vi "Configure.vi"(8 "error in (no error)":errorcluster, 11 "DAQ_QPT_Throlab in":refnum<class "DAQ_QPT_Throlab.lvclass">) -> (0 "error out":errorcluster, 3 "DAQ_QPT_Throlab out":refnum<class "DAQ_QPT_Throlab.lvclass">)   [LabVIEW 2020, in "DAQ_QPT_Throlab.lvlib" / "DAQ_QPT_Throlab.lvclass"]
uses:
  DAQ_QPT_Throlab.lvclass
  E:/Development/DevHardSoftware/MMicroscopyAF/Model/HAL Layer/Component/Device/Device/Device.lvclass
  DAQ_QPT_Throlab.lvclass/DAQ_QPT_Throlab.ctl
  HAL Layer/Component/DAQ/DAQ/DAQ.lvclass
  HAL Layer/Component/Device/Device/Device.lvclass
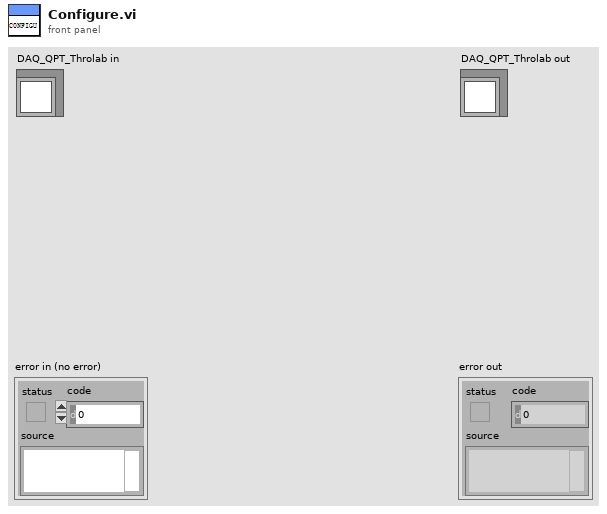
[diagram p1: front panel]
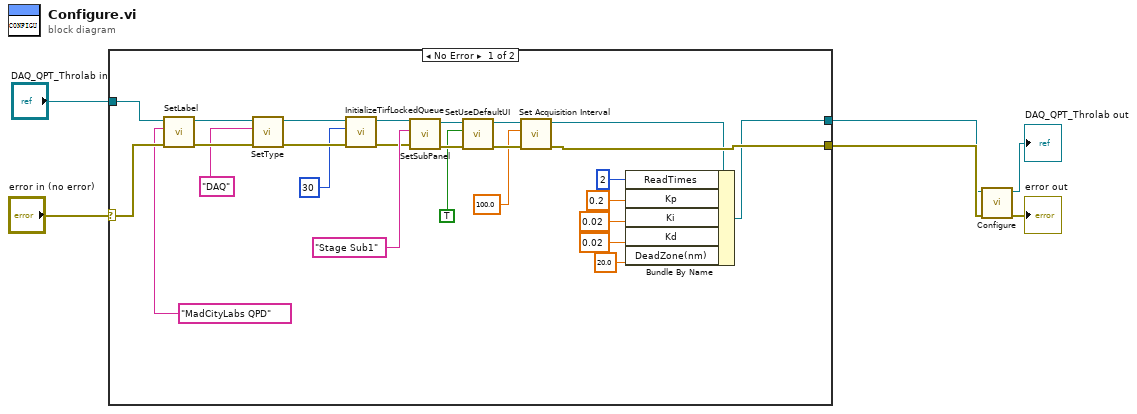
[diagram p0: block diagram]
diagram:
  n1 = case shown="No Error" "error in (no error)" {
    selector: "error in (no error)" -> [w31 w34]
    tunnel: [w20 w34] -> w2
    tunnel: [w12 w33] -> w1
    tunnel: "DAQ_QPT_Throlab in" -> [w32 w33]
    frame No Error {
      n2 = call-dynamic "SetLabel.vi"("error in (no error)"=w31, "Label"="MadCityLabs QPD", "Device in"=w32) -> ("error out"=w28:errorcluster, "Device out"=w29:refnum<class "DAQ_QPT_Throlab.lvclass">)  [unwired: 7 in]
      n3 = call-dynamic "SetType.vi"("error in (no error)"=w28, "Type"="DAQ", "Device in"=w29) -> ("error out"=w26:errorcluster, "Device out"=w16:refnum<class "DAQ_QPT_Throlab.lvclass">)  [unwired: 7 in]
      n4 = call-dynamic "InitializeTirfLockedQueue.vi"("error in (no error)"=w26, "max queue size (-1, unlimited)"=30, "DAQ_QPT_Throlab in"=w16) -> ("error out"=w17:errorcluster, "DAQ_QPT_Throlab out"=w15:refnum<class "DAQ_QPT_Throlab.lvclass">)  [unwired: 7 in]
      n5 = call-dynamic "SetSubPanel.vi"("error in (no error)"=w17, "Sub Panel"="Stage Sub1", "Device in"=w15) -> ("error out"=w25:errorcluster, "Device out"=w22:refnum<class "DAQ_QPT_Throlab.lvclass">)  [unwired: 7 in]
      n6 = call "SetUseDefaultUI.vi"("error in (no error)"=w25, "Use Default UI?"=TRUE, "Device in"=w22) -> ("error out"=w23:errorcluster, "Device out"=w19:refnum<class "DAQ_QPT_Throlab.lvclass">)  [unwired: 7 in]
      n7 = call-dynamic "Set Acquisition Interval.vi"("error in (no error)"=w23, "Interval(ms)"=100.0, "DAQ in"=w19) -> ("error out"=w20:errorcluster, "DAQ out"=w13:refnum<class "DAQ_QPT_Throlab.lvclass">)  [unwired: 7 in]
      n8 = Bundle By Name(cluster=w13, "ReadTimes"=2, "Kp"=0.2 ("PIDParams.Kp"), "Ki"=0.02 ("PIDParams.Ki"), "Kd"=0.02 ("PIDParams.Kd"), "DeadZone(nm)"=20.0 ("PIDParams.DeadZone(nm)")) -> (w12:refnum<class "DAQ_QPT_Throlab.lvclass">)
    }
    frame Error {
    }
  }
  n9 = call-parent "Configure.vi"("error in (no error)"=w2, "Device in"=w1) -> ("error out"=→"error out":errorcluster, "Device out"=→"DAQ_QPT_Throlab out":refnum<class "DAQ_QPT_Throlab.lvclass">)  [unwired: 8 in]
